vi "FeedbackDecode_20200902.vi"() -> ()   [LabVIEW 2016] (continued)
            n1850 = Bundle By Name(cluster=w1875, "ClearWfs"=TRUE, "SelElect"=w1876, "EventStr"=w1891) -> (w1872:T5)
            n1851 = local read "LoopCnt"() -> (w1889:u64)
            n1852 = call "FeedbackDecode_MLComCtrl.vi"("DecodeClustIn"=w1872, "Mode"=T19."SendEvent") -> ("DecodeClustOut"=w1873:T5)  [unwired: 6 in, 3 out]
            n1853 = local write "DecodeClust"(w1873) -> ()
            n1854 = local write "BaseCnt2"(w1889) -> ()
          }
          event Value Change {
            n1855 = event-data() -> ()  [unwired: 1 in, 6 out]
            n1856 = local read "EncodeClust"() -> (w1921:T9)
            n1857 = call "File Dialog2"("pattern (all files)"="StimParams*.txt") -> ("selected path"=w1924:path, "exists"=w1928:bool, "cancelled"=w1927:bool)  [unwired: 11 in, 1 out]
            n1858 = Unbundle By Name(w1921) -> ("SelPreset"=w1923:bool[], "Sel"=w1922:bool[])
            n1859 = local read "DecodeClust"() -> (w1920:T5)
            n1860 = Not(x=w1927) -> (.not. x?=w1929:bool)
            n1861 = And(x=w1928, y=w1929) -> (x .and. y?=w1925:bool)
            n1862 = case shown="True" w1925 {
              tunnel: w1924 -> [_ w1959]
              tunnel: w1923 -> [_ w1962]
              tunnel: w1922 -> [_ w1961]
              tunnel: w1921 -> [w1932 w1960]
              tunnel: w1920 -> [_ w1945]
              frame False {
                n1863 = Bundle By Name(cluster=w1932, "AdjClust.LoadTable"=FALSE) -> (w1931:T9)
                n1864 = local write "EncodeClust"(w1931) -> ()
              }
              frame True {
                n1865 = call-poly <vilib>:"Read Delimited Spreadsheet.vi"("file path (dialog if empty)"=w1959) -> ("all rows"=w1963:string[][])  [unwired: 9 in, 5 out]
                n1866 = Array Size(array=w1962) -> (size(s)=w1965:i32)
                n1867 = Array Size(array=w1961) -> (size(s)=w1968:i32)
                n1868 = Initialize Array(FALSE, w1965) -> (w1969:bool[])
                n1869 = Initialize Array(FALSE, w1968) -> (w1970:bool[])
                n1870 = Bundle By Name(cluster=w1960, "SelPreset"=w1969, "Sel"=w1970, "ParamsTable"=w1963, "AdjClust.LoadTable"=FALSE) -> (w1957:T9)
                n1871 = Path To String(path=w1959) -> (string=w1955:string)
                n1872 = call "FeedbackDecode_UpdateParamsTable.vi"("StimClustIn"=w1957) -> ("StimClustOut"=w1958:T9)  [unwired: 2 in]
                n1873 = call "FeedbackDecode_Params2UEA.vi"("StimClustIn"=w1958) -> ("StimClustOut"=w1940:T9)  [unwired: 2 in]
                n1874 = local read "LoopCnt"() -> (w1949:u64)
                n1875 = local read "NIPTime"() -> (w1938:dbl)
                n1876 = call "FeedbackDecode_BuildStimCmd.vi"("EncodeClustIn"=w1940) -> ("EncodeClustOut"=w1939:T9, "StimCmd"=w1934:string)  [unwired: 1 in]
                n1877 = Search and Replace String(input string=w1955, search string=":", replace string="@" ("replace string (\"\")")) -> (result string=w1942:string)  [unwired: 5 in, 3 out]
                n1878 = Format Into String(w1949) -> (resulting string=w1946:string)  [unwired: 3 in, 1 out]
                n1879 = call-poly "FeedbackDecode_VariablesToString.vi"("Format"="%0.0f", "ValueIn"=w1938, "FieldName"="NIPTime" ("Key Word")) -> ("StringOut"=w1935:string)  [unwired: 4 in]
                n1880 = local write "EncodeClust"(w1939) -> ()
                n1881 = Concatenate Strings("LoadStimParams:SS.EventID=" ("string"), w1946) -> (w1948:string)
                n1882 = Concatenate Strings(w1948, ";", "SS.StimParamsFile='" ("string"), w1942, "';" ("string"), w1934, w1935) -> (w1944:string)
                n1883 = local write "StimCmd"(w1934) -> ()
                n1884 = Bundle By Name(cluster=w1945, "EventStr"=w1944) -> (w1947:T5)
                n1885 = local read "EventParamsFID"() -> (w1953:refnum<file>)
                n1886 = call "FeedbackDecode_MLComCtrl.vi"("DecodeClustIn"=w1947, "Mode"=T19."SendEvent") -> ()  [unwired: 6 in, 4 out]
                n1887 = call "FeedbackDecode_WriteTextEOL.vi"("text"=w1944, "refnum in"=w1953) -> ()  [unwired: 8 in, 2 out]
              }
            }
          }
          event Value Change {
            n1888 = event-data() -> ()  [unwired: 1 in, 6 out]
            n1889 = local read "EncodeClust"() -> (w1972:T9)
            n1890 = call "File Dialog3"("pattern (all files)"="StimPresets*.txt") -> ("selected path"=w1975:path, "exists"=w1979:bool, "cancelled"=w1978:bool)  [unwired: 11 in, 1 out]
            n1891 = Unbundle By Name(w1972) -> ("SelPreset"=w1974:bool[], "Sel"=w1973:bool[])
            n1892 = local read "DecodeClust"() -> (w1971:T5)
            n1893 = Not(x=w1978) -> (.not. x?=w1980:bool)
            n1894 = And(x=w1979, y=w1980) -> (x .and. y?=w1976:bool)
            n1895 = case shown="True" w1976 {
              tunnel: w1975 -> [_ w2011]
              tunnel: w1974 -> [_ w2014]
              tunnel: w1973 -> [_ w2013]
              tunnel: w1972 -> [w1983 w2012]
              tunnel: w1971 -> [_ w1998]
              frame False {
                n1896 = Bundle By Name(cluster=w1983, "AdjClust.LoadTable"=FALSE) -> (w1982:T9)
                n1897 = local write "EncodeClust"(w1982) -> ()
              }
              frame True {
                n1898 = call-poly <vilib>:"Read Delimited Spreadsheet.vi"("file path (dialog if empty)"=w2011) -> ("all rows"=w2015:string[][])  [unwired: 9 in, 5 out]
                n1899 = Array Size(array=w2014) -> (size(s)=w2017:i32)
                n1900 = Array Size(array=w2013) -> (size(s)=w2020:i32)
                n1901 = Initialize Array(FALSE, w2017) -> (w2021:bool[])
                n1902 = Initialize Array(FALSE, w2020) -> (w2022:bool[])
                n1903 = Bundle By Name(cluster=w2012, "SelPreset"=w2021, "Sel"=w2022, "PresetTable"=w2015, "PresetClust.Load"=FALSE ("AdjClust.LoadTable")) -> (w1986:T9)
                n1904 = Path To String(path=w2011) -> (string=w2008:string)
                n1905 = call "FeedbackDecode_UpdatePresetsTable.vi"("StimClustIn"=w1986) -> ("StimClustOut"=w1985:T9)  [unwired: 2 in]
                n1906 = call "FeedbackDecode_UpdateParamsTable.vi"("StimClustIn"=w1985) -> ("StimClustOut"=w2010:T9)  [unwired: 2 in]
                n1907 = call "FeedbackDecode_Params2UEA.vi"("StimClustIn"=w2010) -> ("StimClustOut"=w1993:T9)  [unwired: 2 in]
                n1908 = local read "LoopCnt"() -> (w2002:u64)
                n1909 = local read "NIPTime"() -> (w1991:dbl)
                n1910 = call "FeedbackDecode_BuildStimCmd.vi"("EncodeClustIn"=w1993) -> ("EncodeClustOut"=w1992:T9, "StimCmd"=w1987:string)  [unwired: 1 in]
                n1911 = Search and Replace String(input string=w2008, search string=":", replace string="@" ("replace string (\"\")")) -> (result string=w1995:string)  [unwired: 5 in, 3 out]
                n1912 = Format Into String(w2002) -> (resulting string=w1999:string)  [unwired: 3 in, 1 out]
                n1913 = call-poly "FeedbackDecode_VariablesToString.vi"("Format"="%0.0f", "ValueIn"=w1991, "FieldName"="NIPTime" ("Key Word")) -> ("StringOut"=w1988:string)  [unwired: 4 in]
                n1914 = local write "EncodeClust"(w1992) -> ()
                n1915 = Concatenate Strings("LoadPresets:SS.EventID=" ("string"), w1999) -> (w2001:string)
                n1916 = Concatenate Strings(w2001, ";", "SS.PresetsFile='" ("string"), w1995, "';" ("string"), w1987, w1988) -> (w1997:string)
                n1917 = local write "StimCmd"(w1987) -> ()
                n1918 = Bundle By Name(cluster=w1998, "EventStr"=w1997) -> (w2000:T5)
                n1919 = local read "EventParamsFID"() -> (w2006:refnum<file>)
                n1920 = call "FeedbackDecode_MLComCtrl.vi"("DecodeClustIn"=w2000, "Mode"=T19."SendEvent") -> ()  [unwired: 6 in, 4 out]
                n1921 = call "FeedbackDecode_WriteTextEOL.vi"("text"=w1997, "refnum in"=w2006) -> ()  [unwired: 8 in, 2 out]
              }
            }
          }
          event Value Change {
            n1922 = event-data() -> ()  [unwired: 1 in, 6 out]
            n1923 = local read "DataPath"() -> (w2027:path)
            n1924 = call "File Dialog"("start path"=w2027) -> ("selected path"=w2024:path, "cancelled"=w2026:bool)  [unwired: 11 in, 2 out]
            n1925 = local read "EncodeClust"() -> (w2025:T9)
            n1926 = local read "DecodeClust"() -> (w2023:T5)
            n1927 = case shown="False" w2026 {
              tunnel: w2025 -> [w2038 w2065]
              tunnel: w2024 -> [w2039 _]
              tunnel: w2023 -> [w2029 _]
              frame False {
                w2048 = "_" ("string")
                n1928 = Strip Path(path=w2039) -> (stripped path=w2046:path, name=w2047:string)
                n1929 = Unbundle By Name(w2029) -> ("DataFolder"=w2036:string)
                n1930 = Get Date/Time In Seconds() -> (seconds since 1Jan1904=w2042:timestamp)
                n1931 = Format Date/Time String(time format string (%c)="%H%M%S", seconds (now)=w2042) -> (date/time string=w2044:string)  [unwired: 1 in]
                n1932 = Concatenate Strings("StimParams_" ("name or relative path"), w2036, w2048, w2047, w2048, w2044, ".txt" ("string")) -> (w2045:string)
                n1933 = Unbundle By Name(w2038) -> ("ParamsTable"=w2040:string[][])
                n1934 = Bundle By Name(cluster=w2038, "AdjClust.SaveTable"=FALSE ("Save")) -> (w2058:T9)
                n1935 = Build Path(base path=w2046, name or relative path=w2045) -> (appended path=w2049:path)
                n1936 = call-poly <vilib>:"Write Delimited Spreadsheet.vi"("file path (dialog if empty)"=w2049, "2D data"=w2040) -> ()  [unwired: 12 in, 2 out]
                n1937 = Path To String(path=w2049) -> (string=w2033:string)
                n1938 = local read "LoopCnt"() -> (w2061:u64)
                n1939 = local write "EncodeClust"(w2058) -> ()
                n1940 = Format Into String(w2061) -> (resulting string=w2050:string)  [unwired: 3 in, 1 out]
                n1941 = Search and Replace String(input string=w2033, search string=":", replace string="@" ("replace string (\"\")")) -> (result string=w2031:string)  [unwired: 5 in, 3 out]
                n1942 = local read "NIPTime"() -> (w2055:dbl)
                n1943 = Concatenate Strings("SaveStimParams:SS.EventID=" ("string"), w2050, ";") -> (w2056:string)
                n1944 = local read "EventParamsFID"() -> (w2064:refnum<file>)
                n1945 = call-poly "FeedbackDecode_VariablesToString.vi"("Format"="%0.0f", "ValueIn"=w2055, "FieldName"="NIPTime" ("Key Word")) -> ("StringOut"=w2052:string)  [unwired: 4 in]
                n1946 = Concatenate Strings(w2056, "SS.StimParamsFile='" ("string"), w2031, "';" ("string"), w2052) -> (w2051:string)
                n1947 = call "FeedbackDecode_WriteTextEOL.vi"("text"=w2051, "refnum in"=w2064) -> ()  [unwired: 8 in, 2 out]
                n1948 = Bundle By Name(cluster=w2029, "EventStr"=w2051) -> (w2060:T5)
                n1949 = call "FeedbackDecode_MLComCtrl.vi"("DecodeClustIn"=w2060, "Mode"=T19."SendEvent") -> ()  [unwired: 6 in, 4 out]
              }
              frame True {
                n1950 = Bundle By Name(cluster=w2065, "AdjClust.SaveTable"=FALSE ("Save")) -> (w2067:T9)
                n1951 = local write "EncodeClust"(w2067) -> ()
              }
            }
          }
          event Value Change {
            n1952 = event-data() -> ()  [unwired: 1 in, 6 out]
            n1953 = local read "DataPath"() -> (w2072:path)
            n1954 = call "File Dialog4"("start path"=w2072) -> ("selected path"=w2069:path, "cancelled"=w2071:bool)  [unwired: 11 in, 2 out]
            n1955 = local read "EncodeClust"() -> (w2070:T9)
            n1956 = local read "DecodeClust"() -> (w2068:T5)
            n1957 = case shown="False" w2071 {
              tunnel: w2070 -> [w2083 w2110]
              tunnel: w2069 -> [w2084 _]
              tunnel: w2068 -> [w2074 _]
              frame False {
                w2093 = "_" ("string")
                n1958 = Strip Path(path=w2084) -> (stripped path=w2091:path, name=w2092:string)
                n1959 = Unbundle By Name(w2074) -> ("DataFolder"=w2081:string)
                n1960 = Get Date/Time In Seconds() -> (seconds since 1Jan1904=w2087:timestamp)
                n1961 = Format Date/Time String(time format string (%c)="%H%M%S", seconds (now)=w2087) -> (date/time string=w2089:string)  [unwired: 1 in]
                n1962 = Concatenate Strings("StimPresets_" ("name or relative path"), w2081, w2093, w2092, w2093, w2089, ".txt" ("string")) -> (w2090:string)
                n1963 = Unbundle By Name(w2083) -> ("PresetTable"=w2085:string[][])
                n1964 = Build Path(base path=w2091, name or relative path=w2090) -> (appended path=w2094:path)
                n1965 = Bundle By Name(cluster=w2083, "PresetClust.Save"=FALSE ("Save")) -> (w2103:T9)
                n1966 = call-poly <vilib>:"Write Delimited Spreadsheet.vi"("file path (dialog if empty)"=w2094, "2D data"=w2085) -> ()  [unwired: 12 in, 2 out]
                n1967 = Path To String(path=w2094) -> (string=w2078:string)
                n1968 = local read "LoopCnt"() -> (w2106:u64)
                n1969 = local write "EncodeClust"(w2103) -> ()
                n1970 = Format Into String(w2106) -> (resulting string=w2095:string)  [unwired: 3 in, 1 out]
                n1971 = Search and Replace String(input string=w2078, search string=":", replace string="@" ("replace string (\"\")")) -> (result string=w2076:string)  [unwired: 5 in, 3 out]
                n1972 = local read "NIPTime"() -> (w2100:dbl)
                n1973 = Concatenate Strings("SavePresets:SS.EventID=" ("string"), w2095, ";") -> (w2101:string)
                n1974 = local read "EventParamsFID"() -> (w2109:refnum<file>)
                n1975 = call-poly "FeedbackDecode_VariablesToString.vi"("Format"="%0.0f", "ValueIn"=w2100, "FieldName"="NIPTime" ("Key Word")) -> ("StringOut"=w2097:string)  [unwired: 4 in]
                n1976 = Concatenate Strings(w2101, "SS.PresetsFile='" ("string"), w2076, "';" ("string"), w2097) -> (w2096:string)
                n1977 = call "FeedbackDecode_WriteTextEOL.vi"("text"=w2096, "refnum in"=w2109) -> ()  [unwired: 8 in, 2 out]
                n1978 = Bundle By Name(cluster=w2074, "EventStr"=w2096) -> (w2105:T5)
                n1979 = call "FeedbackDecode_MLComCtrl.vi"("DecodeClustIn"=w2105, "Mode"=T19."SendEvent") -> ()  [unwired: 6 in, 4 out]
              }
              frame True {
                n1980 = Bundle By Name(cluster=w2110, "AdjClust.SaveTable"=FALSE ("Save")) -> (w2112:T9)
                n1981 = local write "EncodeClust"(w2112) -> ()
              }
            }
          }
          event Value Change {
            n1982 = event-data() -> ()  [unwired: 1 in, 6 out]
            n1983 = local read "EncodeClust"() -> (w2117:T9)
            n1984 = call "FeedbackDecode_Params2Preset.vi"("StimClustIn"=w2117) -> ("StimClustOut"=w2116:T9)  [unwired: 2 in]
            n1985 = local read "LoopCnt"() -> (w2126:u64)
            n1986 = call "FeedbackDecode_UpdateParamsTable.vi"("StimClustIn"=w2116) -> ("StimClustOut"=w2115:T9)  [unwired: 2 in]
            n1987 = call "FeedbackDecode_Params2UEA.vi"("StimClustIn"=w2115) -> ("StimClustOut"=w2114:T9)  [unwired: 2 in]
            n1988 = Format Into String(w2126) -> (resulting string=w2118:string)  [unwired: 3 in, 1 out]
            n1989 = local read "NIPTime"() -> (w2122:dbl)
            n1990 = call "FeedbackDecode_BuildStimCmd.vi"("EncodeClustIn"=w2114) -> ("EncodeClustOut"=w2132:T9, "StimCmd"=w2113:string)  [unwired: 1 in]
            n1991 = local read "EventParamsFID"() -> (w2130:refnum<file>)
            n1992 = Concatenate Strings("UpdateStim:SS.EventID=" ("string"), w2118) -> (w2125:string)
            n1993 = call-poly "FeedbackDecode_VariablesToString.vi"("Format"="%0.0f", "ValueIn"=w2122, "FieldName"="NIPTime" ("Key Word")) -> ("StringOut"=w2119:string)  [unwired: 4 in]
            n1994 = local read "DecodeClust"() -> (w2131:T5)
            n1995 = Concatenate Strings(w2125, ";", w2113, w2119) -> (w2124:string)
            n1996 = call "FeedbackDecode_WriteTextEOL.vi"("text"=w2124, "refnum in"=w2130) -> ()  [unwired: 8 in, 2 out]
            n1997 = Bundle By Name(cluster=w2131, "EventStr"=w2124) -> (w2123:T5)
            n1998 = local write "StimCmd"(w2113) -> ()
            n1999 = local write "EncodeClust"(w2132) -> ()
            n2000 = call "FeedbackDecode_MLComCtrl.vi"("DecodeClustIn"=w2123, "Mode"=T19."SendEvent") -> ()  [unwired: 6 in, 4 out]
          }
          event Value Change {
            n2001 = event-data() -> ("NewVal"=w2139:bool[], "OldVal"=w2138:bool[])  [unwired: 1 in, 4 out]
            n2002 = call "FeedbackDecode_UpdateSelPresets.vi"("OldSelIn"=w2138, "NewSelIn"=w2139) -> ("OldSelOut"=w2137:bool[], "NewSelOut"=w2136:bool[])
            n2003 = Exclusive Or(1:w2137, 2:w2136) -> (0:w2134:bool[])
            n2004 = Or Array Elements(Boolean array=w2136) -> (logical OR=w2135:bool)
            n2005 = case shown="False" w2135 {
              tunnel: w2134 -> [w2143 _]
              frame True {
                n2006 = local read "EncodeClust"() -> (w2144:T9)
                n2007 = Bundle By Name(cluster=w2144, "SelPreset"=w2143) -> (w2142:T9)
                n2008 = call "FeedbackDecode_UpdatePresetsTable.vi"("StimClustIn"=w2142) -> ("StimClustOut"=w2147:T9)  [unwired: 2 in]
                n2009 = local read "LoopCnt"() -> (w2156:u64)
                n2010 = call "FeedbackDecode_UpdateParamsTable.vi"("StimClustIn"=w2147) -> ("StimClustOut"=w2146:T9)  [unwired: 2 in]
                n2011 = call "FeedbackDecode_Params2UEA.vi"("StimClustIn"=w2146) -> ("StimClustOut"=w2145:T9)  [unwired: 2 in]
                n2012 = Format Into String(w2156) -> (resulting string=w2148:string)  [unwired: 3 in, 1 out]
                n2013 = local read "NIPTime"() -> (w2152:dbl)
                n2014 = call "FeedbackDecode_BuildStimCmd.vi"("EncodeClustIn"=w2145) -> ("EncodeClustOut"=w2162:T9, "StimCmd"=w2141:string)  [unwired: 1 in]
                n2015 = local read "EventParamsFID"() -> (w2160:refnum<file>)
                n2016 = Concatenate Strings("UpdateStim:SS.EventID=" ("string"), w2148) -> (w2155:string)
                n2017 = call-poly "FeedbackDecode_VariablesToString.vi"("Format"="%0.0f", "ValueIn"=w2152, "FieldName"="NIPTime" ("Key Word")) -> ("StringOut"=w2149:string)  [unwired: 4 in]
                n2018 = local read "DecodeClust"() -> (w2161:T5)
                n2019 = Concatenate Strings(w2155, ";", w2141, w2149) -> (w2154:string)
                n2020 = call "FeedbackDecode_WriteTextEOL.vi"("text"=w2154, "refnum in"=w2160) -> ()  [unwired: 8 in, 2 out]
                n2021 = Bundle By Name(cluster=w2161, "EventStr"=w2154) -> (w2153:T5)
                n2022 = local write "StimCmd"(w2141) -> ()
                n2023 = local write "EncodeClust"(w2162) -> ()
                n2024 = call "FeedbackDecode_MLComCtrl.vi"("DecodeClustIn"=w2153, "Mode"=T19."SendEvent") -> ()  [unwired: 6 in, 4 out]
              }
              frame False {
                n2025 = local read "EncodeClust"() -> (w2165:T9)
                n2026 = Unbundle By Name(w2165) -> ("Sel"=w2167:bool[])
                n2027 = Array Size(array=w2167) -> (size(s)=w2168:i32)
                n2028 = Initialize Array(FALSE, w2168) -> (w2166:bool[])
                n2029 = Bundle By Name(cluster=w2165, "Sel"=w2166) -> (w2164:T9)
                n2030 = local read "LoopCnt"() -> (w2180:u64)
                n2031 = call "FeedbackDecode_UpdateParamsTable.vi"("StimClustIn"=w2164) -> ("StimClustOut"=w2171:T9)  [unwired: 2 in]
                n2032 = call "FeedbackDecode_Params2UEA.vi"("StimClustIn"=w2171) -> ("StimClustOut"=w2170:T9)  [unwired: 2 in]
                n2033 = Format Into String(w2180) -> (resulting string=w2172:string)  [unwired: 3 in, 1 out]
                n2034 = local read "NIPTime"() -> (w2176:dbl)
                n2035 = call "FeedbackDecode_BuildStimCmd.vi"("EncodeClustIn"=w2170) -> ("EncodeClustOut"=w2186:T9, "StimCmd"=w2163:string)  [unwired: 1 in]
                n2036 = local read "EventParamsFID"() -> (w2184:refnum<file>)
                n2037 = Concatenate Strings("UpdateStim:SS.EventID=" ("string"), w2172) -> (w2179:string)
                n2038 = call-poly "FeedbackDecode_VariablesToString.vi"("Format"="%0.0f", "ValueIn"=w2176, "FieldName"="NIPTime" ("Key Word")) -> ("StringOut"=w2173:string)  [unwired: 4 in]
                n2039 = local read "DecodeClust"() -> (w2185:T5)
                n2040 = Concatenate Strings(w2179, ";", w2163, w2173) -> (w2178:string)
                n2041 = call "FeedbackDecode_WriteTextEOL.vi"("text"=w2178, "refnum in"=w2184) -> ()  [unwired: 8 in, 2 out]
                n2042 = Bundle By Name(cluster=w2185, "EventStr"=w2178) -> (w2177:T5)
                n2043 = local write "StimCmd"(w2163) -> ()
                n2044 = local write "EncodeClust"(w2186) -> ()
                n2045 = call "FeedbackDecode_MLComCtrl.vi"("DecodeClustIn"=w2177, "Mode"=T19."SendEvent") -> ()  [unwired: 6 in, 4 out]
              }
            }
          }
          event Value Change {
            n2046 = event-data() -> ()  [unwired: 1 in, 6 out]
            n2047 = local read "EncodeClust"() -> (w2191:T9)
            n2048 = call "FeedbackDecode_UEA2Params.vi"("StimClustIn"=w2191) -> ("StimClustOut"=w2190:T9)  [unwired: 2 in]
            n2049 = local read "LoopCnt"() -> (w2200:u64)
            n2050 = call "FeedbackDecode_UpdateParamsTable.vi"("StimClustIn"=w2190) -> ("StimClustOut"=w2189:T9)  [unwired: 2 in]
            n2051 = call "FeedbackDecode_Params2Preset.vi"("StimClustIn"=w2189) -> ("StimClustOut"=w2188:T9)  [unwired: 2 in]
            n2052 = Format Into String(w2200) -> (resulting string=w2192:string)  [unwired: 3 in, 1 out]
            n2053 = local read "NIPTime"() -> (w2196:dbl)
            n2054 = call "FeedbackDecode_BuildStimCmd.vi"("EncodeClustIn"=w2188) -> ("EncodeClustOut"=w2206:T9, "StimCmd"=w2187:string)  [unwired: 1 in]
            n2055 = local read "EventParamsFID"() -> (w2204:refnum<file>)
            n2056 = Concatenate Strings("UpdateStim:SS.EventID=" ("string"), w2192) -> (w2199:string)
            n2057 = call-poly "FeedbackDecode_VariablesToString.vi"("Format"="%0.0f", "ValueIn"=w2196, "FieldName"="NIPTime" ("Key Word")) -> ("StringOut"=w2193:string)  [unwired: 4 in]
            n2058 = local read "DecodeClust"() -> (w2205:T5)
            n2059 = Concatenate Strings(w2199, ";", w2187, w2193) -> (w2198:string)
            n2060 = call "FeedbackDecode_WriteTextEOL.vi"("text"=w2198, "refnum in"=w2204) -> ()  [unwired: 8 in, 2 out]
            n2061 = Bundle By Name(cluster=w2205, "EventStr"=w2198) -> (w2197:T5)
            n2062 = local write "StimCmd"(w2187) -> ()
            n2063 = local write "EncodeClust"(w2206) -> ()
            n2064 = call "FeedbackDecode_MLComCtrl.vi"("DecodeClustIn"=w2197, "Mode"=T19."SendEvent") -> ()  [unwired: 6 in, 4 out]
          }
          event Value Change {
            n2065 = event-data() -> ()  [unwired: 1 in, 6 out]
            n2066 = local read "EncodeClust"() -> (w2213:T9)
            n2067 = call "FeedbackDecode_AdjParamsTable.vi"("StimClustIn"=w2213, "Mode"=enum16{"Set", "Add", "Sub"}."Set") -> ("StimClustOut"=w2211:T9)  [unwired: 1 in]
            n2068 = Bundle By Name(cluster=w2211, "AdjClust.Set"=FALSE) -> (w2209:T9)
            n2069 = local read "LoopCnt"() -> (w2223:u64)
            n2070 = call "FeedbackDecode_Params2Preset.vi"("StimClustIn"=w2209) -> ("StimClustOut"=w2214:T9)  [unwired: 2 in]
            n2071 = Format Into String(w2223) -> (resulting string=w2215:string)  [unwired: 3 in, 1 out]
            n2072 = local read "NIPTime"() -> (w2219:dbl)
            n2073 = call "FeedbackDecode_BuildStimCmd.vi"("EncodeClustIn"=w2214) -> ("EncodeClustOut"=w2229:T9, "StimCmd"=w2208:string)  [unwired: 1 in]
            n2074 = local read "EventParamsFID"() -> (w2227:refnum<file>)
            n2075 = Concatenate Strings("UpdateStim:SS.EventID=" ("string"), w2215) -> (w2222:string)
            n2076 = call-poly "FeedbackDecode_VariablesToString.vi"("Format"="%0.0f", "ValueIn"=w2219, "FieldName"="NIPTime" ("Key Word")) -> ("StringOut"=w2216:string)  [unwired: 4 in]
            n2077 = local read "DecodeClust"() -> (w2228:T5)
            n2078 = Concatenate Strings(w2222, ";", w2208, w2216) -> (w2221:string)
            n2079 = call "FeedbackDecode_WriteTextEOL.vi"("text"=w2221, "refnum in"=w2227) -> ()  [unwired: 8 in, 2 out]
            n2080 = Bundle By Name(cluster=w2228, "EventStr"=w2221) -> (w2220:T5)
            n2081 = local write "StimCmd"(w2208) -> ()
            n2082 = local write "EncodeClust"(w2229) -> ()
            n2083 = call "FeedbackDecode_MLComCtrl.vi"("DecodeClustIn"=w2220, "Mode"=T19."SendEvent") -> ()  [unwired: 6 in, 4 out]
          }
          event Value Change {
            n2084 = event-data() -> ()  [unwired: 1 in, 6 out]
            n2085 = local read "EncodeClust"() -> (w2236:T9)
            n2086 = call "FeedbackDecode_AdjParamsTable.vi"("StimClustIn"=w2236, "Mode"=enum16{"Set", "Add", "Sub"}."Add") -> ("StimClustOut"=w2234:T9)  [unwired: 1 in]
            n2087 = Bundle By Name(cluster=w2234, "AdjClust.Add"=FALSE ("AdjClust.Set")) -> (w2232:T9)
            n2088 = local read "LoopCnt"() -> (w2246:u64)
            n2089 = call "FeedbackDecode_Params2Preset.vi"("StimClustIn"=w2232) -> ("StimClustOut"=w2237:T9)  [unwired: 2 in]
            n2090 = Format Into String(w2246) -> (resulting string=w2238:string)  [unwired: 3 in, 1 out]
            n2091 = local read "NIPTime"() -> (w2242:dbl)
            n2092 = call "FeedbackDecode_BuildStimCmd.vi"("EncodeClustIn"=w2237) -> ("EncodeClustOut"=w2252:T9, "StimCmd"=w2231:string)  [unwired: 1 in]
            n2093 = local read "EventParamsFID"() -> (w2250:refnum<file>)
            n2094 = Concatenate Strings("UpdateStim:SS.EventID=" ("string"), w2238) -> (w2245:string)
            n2095 = call-poly "FeedbackDecode_VariablesToString.vi"("Format"="%0.0f", "ValueIn"=w2242, "FieldName"="NIPTime" ("Key Word")) -> ("StringOut"=w2239:string)  [unwired: 4 in]
            n2096 = local read "DecodeClust"() -> (w2251:T5)
            n2097 = Concatenate Strings(w2245, ";", w2231, w2239) -> (w2244:string)
            n2098 = call "FeedbackDecode_WriteTextEOL.vi"("text"=w2244, "refnum in"=w2250) -> ()  [unwired: 8 in, 2 out]
            n2099 = Bundle By Name(cluster=w2251, "EventStr"=w2244) -> (w2243:T5)
            n2100 = local write "StimCmd"(w2231) -> ()
            n2101 = local write "EncodeClust"(w2252) -> ()
            n2102 = call "FeedbackDecode_MLComCtrl.vi"("DecodeClustIn"=w2243, "Mode"=T19."SendEvent") -> ()  [unwired: 6 in, 4 out]
          }
          event Value Change {
            n2103 = event-data() -> ()  [unwired: 1 in, 6 out]
            n2104 = local read "EncodeClust"() -> (w2259:T9)
            n2105 = call "FeedbackDecode_AdjParamsTable.vi"("StimClustIn"=w2259, "Mode"=enum16{"Set", "Add", "Sub"}."Sub") -> ("StimClustOut"=w2257:T9)  [unwired: 1 in]
            n2106 = Bundle By Name(cluster=w2257, "AdjClust.Sub"=FALSE ("AdjClust.Set")) -> (w2255:T9)
            n2107 = local read "LoopCnt"() -> (w2269:u64)
            n2108 = call "FeedbackDecode_Params2Preset.vi"("StimClustIn"=w2255) -> ("StimClustOut"=w2260:T9)  [unwired: 2 in]
            n2109 = Format Into String(w2269) -> (resulting string=w2261:string)  [unwired: 3 in, 1 out]
            n2110 = local read "NIPTime"() -> (w2265:dbl)
            n2111 = call "FeedbackDecode_BuildStimCmd.vi"("EncodeClustIn"=w2260) -> ("EncodeClustOut"=w2275:T9, "StimCmd"=w2254:string)  [unwired: 1 in]
            n2112 = local read "EventParamsFID"() -> (w2273:refnum<file>)
            n2113 = Concatenate Strings("UpdateStim:SS.EventID=" ("string"), w2261) -> (w2268:string)
            n2114 = call-poly "FeedbackDecode_VariablesToString.vi"("Format"="%0.0f", "ValueIn"=w2265, "FieldName"="NIPTime" ("Key Word")) -> ("StringOut"=w2262:string)  [unwired: 4 in]
            n2115 = local read "DecodeClust"() -> (w2274:T5)
            n2116 = Concatenate Strings(w2268, ";", w2254, w2262) -> (w2267:string)
            n2117 = call "FeedbackDecode_WriteTextEOL.vi"("text"=w2267, "refnum in"=w2273) -> ()  [unwired: 8 in, 2 out]
            n2118 = Bundle By Name(cluster=w2274, "EventStr"=w2267) -> (w2266:T5)
            n2119 = local write "StimCmd"(w2254) -> ()
            n2120 = local write "EncodeClust"(w2275) -> ()
            n2121 = call "FeedbackDecode_MLComCtrl.vi"("DecodeClustIn"=w2266, "Mode"=T19."SendEvent") -> ()  [unwired: 6 in, 4 out]
          }
          event Value Change {
            n2122 = event-data() -> ()  [unwired: 1 in, 6 out]
            n2123 = local read "EncodeClust"() -> (w2289:T9)
            n2124 = Unbundle By Name(w2289) -> ("Sel"=w2282:bool[], "ParamsTable"=w2283:string[][], "SelPreset"=w2287:bool[])
            n2125 = while {
              shift-right: [w2315] -> w2281
              shift-left: w2282 -> [w2314]
              shift-right: [w2310] -> w2280
              shift-left: w2283 -> [w2311]
              stop <- w2308 stop-if-true
              n2126 = Search 1D Array(1D array=w2314, element=TRUE) -> (index of element=w2309:i32)  [unwired: 1 in]
              n2127 = Less Than 0?(x=w2309) -> (x < 0?=w2308:bool)
              n2128 = Delete From Array(array=w2314, length=1, index=w2309) -> (array with subset deleted=w2315:bool[])  [unwired: 1 out]
              n2129 = Delete From Array(array=w2311, length=1, index (row)=w2309) -> (array with subset deleted=w2310:string[][])  [unwired: 1 in, 1 out]
            }
            n2130 = Array Size(array=w2287) -> (size(s)=w2285:i32)
            n2131 = Initialize Array(FALSE, w2285) -> (w2288:bool[])
            n2132 = Bundle By Name(cluster=w2289, "Sel"=w2281, "ParamsTable"=w2280, "AdjClust.DeleteSel"=FALSE, "SelPreset"=w2288) -> (w2279:T9)
            n2133 = local read "LoopCnt"() -> (w2299:u64)
            n2134 = call "FeedbackDecode_UpdateParamsTable.vi"("StimClustIn"=w2279) -> ("StimClustOut"=w2278:T9)  [unwired: 2 in]
            n2135 = call "FeedbackDecode_Params2UEA.vi"("StimClustIn"=w2278) -> ("StimClustOut"=w2290:T9)  [unwired: 2 in]
            n2136 = Format Into String(w2299) -> (resulting string=w2291:string)  [unwired: 3 in, 1 out]
            n2137 = local read "NIPTime"() -> (w2295:dbl)
            n2138 = call "FeedbackDecode_BuildStimCmd.vi"("EncodeClustIn"=w2290) -> ("EncodeClustOut"=w2305:T9, "StimCmd"=w2277:string)  [unwired: 1 in]
            n2139 = local read "EventParamsFID"() -> (w2303:refnum<file>)
            n2140 = Concatenate Strings("DelStimParam:SS.EventID=" ("string"), w2291) -> (w2298:string)
            n2141 = call-poly "FeedbackDecode_VariablesToString.vi"("Format"="%0.0f", "ValueIn"=w2295, "FieldName"="NIPTime" ("Key Word")) -> ("StringOut"=w2292:string)  [unwired: 4 in]
            n2142 = local read "DecodeClust"() -> (w2304:T5)
            n2143 = Concatenate Strings(w2298, ";", w2277, w2292) -> (w2297:string)
            n2144 = call "FeedbackDecode_WriteTextEOL.vi"("text"=w2297, "refnum in"=w2303) -> ()  [unwired: 8 in, 2 out]
            n2145 = Bundle By Name(cluster=w2304, "EventStr"=w2297) -> (w2296:T5)
            n2146 = local write "StimCmd"(w2277) -> ()
            n2147 = local write "EncodeClust"(w2305) -> ()
            n2148 = call "FeedbackDecode_MLComCtrl.vi"("DecodeClustIn"=w2296, "Mode"=T19."SendEvent") -> ()  [unwired: 6 in, 4 out]
          }
          event Value Change {
            n2149 = event-data() -> ()  [unwired: 1 in, 6 out]
            n2150 = local read "EncodeClust"() -> (w2329:T9)
            n2151 = Unbundle By Name(w2329) -> ("SelPreset"=w2322:bool[], "PresetTable"=w2323:string[][], "Sel"=w2327:bool[])
            n2152 = while {
              shift-right: [w2355] -> w2321
              shift-left: w2322 -> [w2354]
              shift-right: [w2350] -> w2320
              shift-left: w2323 -> [w2351]
              stop <- w2348 stop-if-true
              n2153 = Search 1D Array(1D array=w2354, element=TRUE) -> (index of element=w2349:i32)  [unwired: 1 in]
              n2154 = Less Than 0?(x=w2349) -> (x < 0?=w2348:bool)
              n2155 = Delete From Array(array=w2354, length=1, index=w2349) -> (array with subset deleted=w2355:bool[])  [unwired: 1 out]
              n2156 = Delete From Array(array=w2351, length=1, index (row)=w2349) -> (array with subset deleted=w2350:string[][])  [unwired: 1 in, 1 out]
            }
            n2157 = Array Size(array=w2327) -> (size(s)=w2325:i32)
            n2158 = Initialize Array(FALSE, w2325) -> (w2328:bool[])
            n2159 = Bundle By Name(cluster=w2329, "SelPreset"=w2321, "PresetTable"=w2320, "PresetClust.Del"=FALSE ("AdjClust.DeleteSel"), "Sel"=w2328) -> (w2317:T9)
            n2160 = call "FeedbackDecode_UpdatePresetsTable.vi"("StimClustIn"=w2317) -> ("StimClustOut"=w2316:T9)  [unwired: 2 in]
            n2161 = local read "LoopCnt"() -> (w2339:u64)
            n2162 = call "FeedbackDecode_UpdateParamsTable.vi"("StimClustIn"=w2316) -> ("StimClustOut"=w2319:T9)  [unwired: 2 in]
            n2163 = call "FeedbackDecode_Params2UEA.vi"("StimClustIn"=w2319) -> ("StimClustOut"=w2330:T9)  [unwired: 2 in]
            n2164 = Format Into String(w2339) -> (resulting string=w2331:string)  [unwired: 3 in, 1 out]
            n2165 = local read "NIPTime"() -> (w2335:dbl)
            n2166 = call "FeedbackDecode_BuildStimCmd.vi"("EncodeClustIn"=w2330) -> ("EncodeClustOut"=w2345:T9, "StimCmd"=w2318:string)  [unwired: 1 in]
            n2167 = local read "EventParamsFID"() -> (w2343:refnum<file>)
            n2168 = Concatenate Strings("DelPreset:SS.EventID=" ("string"), w2331) -> (w2338:string)
            n2169 = call-poly "FeedbackDecode_VariablesToString.vi"("Format"="%0.0f", "ValueIn"=w2335, "FieldName"="NIPTime" ("Key Word")) -> ("StringOut"=w2332:string)  [unwired: 4 in]
            n2170 = local read "DecodeClust"() -> (w2344:T5)
            n2171 = Concatenate Strings(w2338, ";", w2318, w2332) -> (w2337:string)
            n2172 = call "FeedbackDecode_WriteTextEOL.vi"("text"=w2337, "refnum in"=w2343) -> ()  [unwired: 8 in, 2 out]
            n2173 = Bundle By Name(cluster=w2344, "EventStr"=w2337) -> (w2336:T5)
            n2174 = local write "StimCmd"(w2318) -> ()
            n2175 = local write "EncodeClust"(w2345) -> ()
            n2176 = call "FeedbackDecode_MLComCtrl.vi"("DecodeClustIn"=w2336, "Mode"=T19."SendEvent") -> ()  [unwired: 6 in, 4 out]
          }
          event Value Change {
            n2177 = event-data() -> ()  [unwired: 1 in, 6 out]
            n2178 = local read "EncodeClust"() -> (w2366:T9)
            n2179 = Unbundle By Name(w2366) -> ("SelPreset"=w2362:bool[])
            n2180 = Array Size(array=w2362) -> (size(s)=w2364:i32)
            n2181 = Initialize Array(FALSE, w2364) -> (w2365:bool[])
            n2182 = Bundle By Name(cluster=w2366, "ParamsTable"=string[][] [], "Sel"=bool[] [], "UEAArray"=T25 [{"Boolean 1"=FALSE, "Boolean 2"=FALSE, "Boolean 3"=FALSE, "Boolean 4"=FALSE, "Boolean 5"=FALSE, "Boolean 6"=FALSE, "Boolean 7"=FALSE, "Boolean 8"=FALSE, "Boolean 9"=FALSE, "Boolean 10"=FALSE, "Boolean 11"=FALSE, "Boolean 12"=FALSE, "Boolean 13"=FALSE, "Boolean 14"=FALSE, "Boolean 15"=FALSE, "Boolean 16"=FALSE, "Boolean 17"=FALSE, "Boolean 18"=FALSE, "Boolean 19"=FALSE, "Boolean 20"=FALSE, "Boolean 21"=FALSE, "Boolean 22"=FALSE, "Boolean 23"=FALSE, "Boolean 24"=FALSE, "Boolean 25"=FALSE, "Boolean 26"=FALSE, "Boolean 27"=FALSE, "Boolean 28"=FALSE, "Boolean 29"=FALSE, "Boolean 30"=FALSE, "Boolean 31"=FALSE, "Boolean 32"=FALSE, "Boolean 33"=FALSE, "Boolean 34"=FALSE, "Boolean 35"=FALSE, "Boolean 36"=FALSE, "Boolean 37"=FALSE, "Boolean 38"=FALSE, "Boolean 39"=FALSE, "Boolean 40"=FALSE, "Boolean 41"=FALSE, "Boolean 42"=FALSE, "Boolean 43"=FALSE, "Boolean 44"=FALSE, "Boolean 45"=FALSE, "Boolean 46"=FALSE, "Boolean 47"=FALSE, "Boolean 48"=FALSE, "Boolean 49"=FALSE, "Boolean 50"=FALSE, "Boolean 51"=FALSE, "Boolean 52"=FALSE, "Boolean 53"=FALSE, "Boolean 54"=FALSE, "Boolean 55"=FALSE, "Boolean 56"=FALSE, "Boolean 57"=FALSE, "Boolean 58"=FALSE, "Boolean 59"=FALSE, "Boolean 60"=FALSE, "Boolean 61"=FALSE, "Boolean 62"=FALSE, "Boolean 63"=FALSE, "Boolean 64"=FALSE, "Boolean 65"=FALSE, "Boolean 66"=FALSE, "Boolean 67"=FALSE, "Boolean 68"=FALSE, "Boolean 69"=FALSE, "Boolean 70"=FALSE, "Boolean 71"=FALSE, "Boolean 72"=FALSE, "Boolean 73"=FALSE, "Boolean 74"=FALSE, "Boolean 75"=FALSE, "Boolean 76"=FALSE, "Boolean 77"=FALSE, "Boolean 78"=FALSE, "Boolean 79"=FALSE, "Boolean 80"=FALSE, "Boolean 81"=FALSE, "Boolean 82"=FALSE, "Boolean 83"=FALSE, "Boolean 84"=FALSE, "Boolean 85"=FALSE, "Boolean 86"=FALSE, "Boolean 87"=FALSE, "Boolean 88"=FALSE, "Boolean 89"=FALSE, "Boolean 90"=FALSE, "Boolean 91"=FALSE, "Boolean 92"=FALSE, "Boolean 93"=FALSE, "Boolean 94"=FALSE, "Boolean 95"=FALSE, "Boolean 96"=FALSE, "Boolean 97"=FALSE, "Boolean 98"=FALSE, "Boolean 99"=FALSE, "Boolean 100"=FALSE}, {"Boolean 1"=FALSE, "Boolean 2"=FALSE, "Boolean 3"=FALSE, "Boolean 4"=FALSE, "Boolean 5"=FALSE, "Boolean 6"=FALSE, "Boolean 7"=FALSE, "Boolean 8"=FALSE, "Boolean 9"=FALSE, "Boolean 10"=FALSE, "Boolean 11"=FALSE, "Boolean 12"=FALSE, "Boolean 13"=FALSE, "Boolean 14"=FALSE, "Boolean 15"=FALSE, "Boolean 16"=FALSE, "Boolean 17"=FALSE, "Boolean 18"=FALSE, "Boolean 19"=FALSE, "Boolean 20"=FALSE, "Boolean 21"=FALSE, "Boolean 22"=FALSE, "Boolean 23"=FALSE, "Boolean 24"=FALSE, "Boolean 25"=FALSE, "Boolean 26"=FALSE, "Boolean 27"=FALSE, "Boolean 28"=FALSE, "Boolean 29"=FALSE, "Boolean 30"=FALSE, "Boolean 31"=FALSE, "Boolean 32"=FALSE, "Boolean 33"=FALSE, "Boolean 34"=FALSE, "Boolean 35"=FALSE, "Boolean 36"=FALSE, "Boolean 37"=FALSE, "Boolean 38"=FALSE, "Boolean 39"=FALSE, "Boolean 40"=FALSE, "Boolean 41"=FALSE, "Boolean 42"=FALSE, "Boolean 43"=FALSE, "Boolean 44"=FALSE, "Boolean 45"=FALSE, "Boolean 46"=FALSE, "Boolean 47"=FALSE, "Boolean 48"=FALSE, "Boolean 49"=FALSE, "Boolean 50"=FALSE, "Boolean 51"=FALSE, "Boolean 52"=FALSE, "Boolean 53"=FALSE, "Boolean 54"=FALSE, "Boolean 55"=FALSE, "Boolean 56"=FALSE, "Boolean 57"=FALSE, "Boolean 58"=FALSE, "Boolean 59"=FALSE, "Boolean 60"=FALSE, "Boolean 61"=FALSE, "Boolean 62"=FALSE, "Boolean 63"=FALSE, "Boolean 64"=FALSE, "Boolean 65"=FALSE, "Boolean 66"=FALSE, "Boolean 67"=FALSE, "Boolean 68"=FALSE, "Boolean 69"=FALSE, "Boolean 70"=FALSE, "Boolean 71"=FALSE, "Boolean 72"=FALSE, "Boolean 73"=FALSE, "Boolean 74"=FALSE, "Boolean 75"=FALSE, "Boolean 76"=FALSE, "Boolean 77"=FALSE, "Boolean 78"=FALSE, "Boolean 79"=FALSE, "Boolean 80"=FALSE, "Boolean 81"=FALSE, "Boolean 82"=FALSE, "Boolean 83"=FALSE, "Boolean 84"=FALSE, "Boolean 85"=FALSE, "Boolean 86"=FALSE, "Boolean 87"=FALSE, "Boolean 88"=FALSE, "Boolean 89"=FALSE, "Boolean 90"=FALSE, "Boolean 91"=FALSE, "Boolean 92"=FALSE, "Boolean 93"=FALSE, "Boolean 94"=FALSE, "Boolean 95"=FALSE, "Boolean 96"=FALSE, "Boolean 97"=FALSE, "Boolean 98"=FALSE, "Boolean 99"=FALSE, "Boolean 100"=FALSE}], "AdjClust.ClearTable"=FALSE, "SelPreset"=w2365) -> (w2357:T9)
            n2183 = local read "LoopCnt"() -> (w2377:u64)
            n2184 = call "FeedbackDecode_UpdateParamsTable.vi"("StimClustIn"=w2357) -> ("StimClustOut"=w2367:T9)  [unwired: 2 in]
            n2185 = call "FeedbackDecode_Params2UEA.vi"("StimClustIn"=w2367) -> ("StimClustOut"=w2368:T9)  [unwired: 2 in]
            n2186 = Format Into String(w2377) -> (resulting string=w2369:string)  [unwired: 3 in, 1 out]
            n2187 = local read "NIPTime"() -> (w2373:dbl)
            n2188 = call "FeedbackDecode_BuildStimCmd.vi"("EncodeClustIn"=w2368) -> ("EncodeClustOut"=w2383:T9, "StimCmd"=w2356:string)  [unwired: 1 in]
            n2189 = local read "EventParamsFID"() -> (w2381:refnum<file>)
            n2190 = Concatenate Strings("ClearStimParams:SS.EventID=" ("string"), w2369) -> (w2376:string)
            n2191 = call-poly "FeedbackDecode_VariablesToString.vi"("Format"="%0.0f", "ValueIn"=w2373, "FieldName"="NIPTime" ("Key Word")) -> ("StringOut"=w2370:string)  [unwired: 4 in]
            n2192 = local read "DecodeClust"() -> (w2382:T5)
            n2193 = Concatenate Strings(w2376, ";", w2356, w2370) -> (w2375:string)
            n2194 = call "FeedbackDecode_WriteTextEOL.vi"("text"=w2375, "refnum in"=w2381) -> ()  [unwired: 8 in, 2 out]
            n2195 = Bundle By Name(cluster=w2382, "EventStr"=w2375) -> (w2374:T5)
            n2196 = local write "StimCmd"(w2356) -> ()
            n2197 = local write "EncodeClust"(w2383) -> ()
            n2198 = call "FeedbackDecode_MLComCtrl.vi"("DecodeClustIn"=w2374, "Mode"=T19."SendEvent") -> ()  [unwired: 6 in, 4 out]
          }
          event Value Change {
            n2199 = event-data() -> ()  [unwired: 1 in, 6 out]
            n2200 = local read "EncodeClust"() -> (w2396:T9)
            n2201 = Unbundle By Name(w2396) -> ("Sel"=w2392:bool[])
            n2202 = Array Size(array=w2392) -> (size(s)=w2394:i32)
            n2203 = Initialize Array(FALSE, w2394) -> (w2395:bool[])
            n2204 = Bundle By Name(cluster=w2396, "PresetTable"=string[][] [] ("ParamsTable"), "SelPreset"=bool[] [] ("Sel"), "UEAArray"=T25 [{"Boolean 1"=FALSE, "Boolean 2"=FALSE, "Boolean 3"=FALSE, "Boolean 4"=FALSE, "Boolean 5"=FALSE, "Boolean 6"=FALSE, "Boolean 7"=FALSE, "Boolean 8"=FALSE, "Boolean 9"=FALSE, "Boolean 10"=FALSE, "Boolean 11"=FALSE, "Boolean 12"=FALSE, "Boolean 13"=FALSE, "Boolean 14"=FALSE, "Boolean 15"=FALSE, "Boolean 16"=FALSE, "Boolean 17"=FALSE, "Boolean 18"=FALSE, "Boolean 19"=FALSE, "Boolean 20"=FALSE, "Boolean 21"=FALSE, "Boolean 22"=FALSE, "Boolean 23"=FALSE, "Boolean 24"=FALSE, "Boolean 25"=FALSE, "Boolean 26"=FALSE, "Boolean 27"=FALSE, "Boolean 28"=FALSE, "Boolean 29"=FALSE, "Boolean 30"=FALSE, "Boolean 31"=FALSE, "Boolean 32"=FALSE, "Boolean 33"=FALSE, "Boolean 34"=FALSE, "Boolean 35"=FALSE, "Boolean 36"=FALSE, "Boolean 37"=FALSE, "Boolean 38"=FALSE, "Boolean 39"=FALSE, "Boolean 40"=FALSE, "Boolean 41"=FALSE, "Boolean 42"=FALSE, "Boolean 43"=FALSE, "Boolean 44"=FALSE, "Boolean 45"=FALSE, "Boolean 46"=FALSE, "Boolean 47"=FALSE, "Boolean 48"=FALSE, "Boolean 49"=FALSE, "Boolean 50"=FALSE, "Boolean 51"=FALSE, "Boolean 52"=FALSE, "Boolean 53"=FALSE, "Boolean 54"=FALSE, "Boolean 55"=FALSE, "Boolean 56"=FALSE, "Boolean 57"=FALSE, "Boolean 58"=FALSE, "Boolean 59"=FALSE, "Boolean 60"=FALSE, "Boolean 61"=FALSE, "Boolean 62"=FALSE, "Boolean 63"=FALSE, "Boolean 64"=FALSE, "Boolean 65"=FALSE, "Boolean 66"=FALSE, "Boolean 67"=FALSE, "Boolean 68"=FALSE, "Boolean 69"=FALSE, "Boolean 70"=FALSE, "Boolean 71"=FALSE, "Boolean 72"=FALSE, "Boolean 73"=FALSE, "Boolean 74"=FALSE, "Boolean 75"=FALSE, "Boolean 76"=FALSE, "Boolean 77"=FALSE, "Boolean 78"=FALSE, "Boolean 79"=FALSE, "Boolean 80"=FALSE, "Boolean 81"=FALSE, "Boolean 82"=FALSE, "Boolean 83"=FALSE, "Boolean 84"=FALSE, "Boolean 85"=FALSE, "Boolean 86"=FALSE, "Boolean 87"=FALSE, "Boolean 88"=FALSE, "Boolean 89"=FALSE, "Boolean 90"=FALSE, "Boolean 91"=FALSE, "Boolean 92"=FALSE, "Boolean 93"=FALSE, "Boolean 94"=FALSE, "Boolean 95"=FALSE, "Boolean 96"=FALSE, "Boolean 97"=FALSE, "Boolean 98"=FALSE, "Boolean 99"=FALSE, "Boolean 100"=FALSE}, {"Boolean 1"=FALSE, "Boolean 2"=FALSE, "Boolean 3"=FALSE, "Boolean 4"=FALSE, "Boolean 5"=FALSE, "Boolean 6"=FALSE, "Boolean 7"=FALSE, "Boolean 8"=FALSE, "Boolean 9"=FALSE, "Boolean 10"=FALSE, "Boolean 11"=FALSE, "Boolean 12"=FALSE, "Boolean 13"=FALSE, "Boolean 14"=FALSE, "Boolean 15"=FALSE, "Boolean 16"=FALSE, "Boolean 17"=FALSE, "Boolean 18"=FALSE, "Boolean 19"=FALSE, "Boolean 20"=FALSE, "Boolean 21"=FALSE, "Boolean 22"=FALSE, "Boolean 23"=FALSE, "Boolean 24"=FALSE, "Boolean 25"=FALSE, "Boolean 26"=FALSE, "Boolean 27"=FALSE, "Boolean 28"=FALSE, "Boolean 29"=FALSE, "Boolean 30"=FALSE, "Boolean 31"=FALSE, "Boolean 32"=FALSE, "Boolean 33"=FALSE, "Boolean 34"=FALSE, "Boolean 35"=FALSE, "Boolean 36"=FALSE, "Boolean 37"=FALSE, "Boolean 38"=FALSE, "Boolean 39"=FALSE, "Boolean 40"=FALSE, "Boolean 41"=FALSE, "Boolean 42"=FALSE, "Boolean 43"=FALSE, "Boolean 44"=FALSE, "Boolean 45"=FALSE, "Boolean 46"=FALSE, "Boolean 47"=FALSE, "Boolean 48"=FALSE, "Boolean 49"=FALSE, "Boolean 50"=FALSE, "Boolean 51"=FALSE, "Boolean 52"=FALSE, "Boolean 53"=FALSE, "Boolean 54"=FALSE, "Boolean 55"=FALSE, "Boolean 56"=FALSE, "Boolean 57"=FALSE, "Boolean 58"=FALSE, "Boolean 59"=FALSE, "Boolean 60"=FALSE, "Boolean 61"=FALSE, "Boolean 62"=FALSE, "Boolean 63"=FALSE, "Boolean 64"=FALSE, "Boolean 65"=FALSE, "Boolean 66"=FALSE, "Boolean 67"=FALSE, "Boolean 68"=FALSE, "Boolean 69"=FALSE, "Boolean 70"=FALSE, "Boolean 71"=FALSE, "Boolean 72"=FALSE, "Boolean 73"=FALSE, "Boolean 74"=FALSE, "Boolean 75"=FALSE, "Boolean 76"=FALSE, "Boolean 77"=FALSE, "Boolean 78"=FALSE, "Boolean 79"=FALSE, "Boolean 80"=FALSE, "Boolean 81"=FALSE, "Boolean 82"=FALSE, "Boolean 83"=FALSE, "Boolean 84"=FALSE, "Boolean 85"=FALSE, "Boolean 86"=FALSE, "Boolean 87"=FALSE, "Boolean 88"=FALSE, "Boolean 89"=FALSE, "Boolean 90"=FALSE, "Boolean 91"=FALSE, "Boolean 92"=FALSE, "Boolean 93"=FALSE, "Boolean 94"=FALSE, "Boolean 95"=FALSE, "Boolean 96"=FALSE, "Boolean 97"=FALSE, "Boolean 98"=FALSE, "Boolean 99"=FALSE, "Boolean 100"=FALSE}], "PresetClust.Clear"=FALSE ("AdjClust.ClearTable"), "Sel"=w2395) -> (w2386:T9)
            n2205 = call "FeedbackDecode_UpdatePresetsTable.vi"("StimClustIn"=w2386) -> ("StimClustOut"=w2385:T9)  [unwired: 2 in]
            n2206 = local read "LoopCnt"() -> (w2407:u64)
            n2207 = call "FeedbackDecode_UpdateParamsTable.vi"("StimClustIn"=w2385) -> ("StimClustOut"=w2397:T9)  [unwired: 2 in]
            n2208 = call "FeedbackDecode_Params2UEA.vi"("StimClustIn"=w2397) -> ("StimClustOut"=w2398:T9)  [unwired: 2 in]
            n2209 = Format Into String(w2407) -> (resulting string=w2399:string)  [unwired: 3 in, 1 out]
            n2210 = local read "NIPTime"() -> (w2403:dbl)
            n2211 = call "FeedbackDecode_BuildStimCmd.vi"("EncodeClustIn"=w2398) -> ("EncodeClustOut"=w2413:T9, "StimCmd"=w2387:string)  [unwired: 1 in]
            n2212 = local read "EventParamsFID"() -> (w2411:refnum<file>)
            n2213 = Concatenate Strings("ClearPresets:SS.EventID=" ("string"), w2399) -> (w2406:string)
            n2214 = call-poly "FeedbackDecode_VariablesToString.vi"("Format"="%0.0f", "ValueIn"=w2403, "FieldName"="NIPTime" ("Key Word")) -> ("StringOut"=w2400:string)  [unwired: 4 in]
            n2215 = local read "DecodeClust"() -> (w2412:T5)
            n2216 = Concatenate Strings(w2406, ";", w2387, w2400) -> (w2405:string)
            n2217 = call "FeedbackDecode_WriteTextEOL.vi"("text"=w2405, "refnum in"=w2411) -> ()  [unwired: 8 in, 2 out]
            n2218 = Bundle By Name(cluster=w2412, "EventStr"=w2405) -> (w2404:T5)
            n2219 = local write "StimCmd"(w2387) -> ()
            n2220 = local write "EncodeClust"(w2413) -> ()
            n2221 = call "FeedbackDecode_MLComCtrl.vi"("DecodeClustIn"=w2404, "Mode"=T19."SendEvent") -> ()  [unwired: 6 in, 4 out]
          }
          event Value Change {
            n2222 = event-data() -> ()  [unwired: 1 in, 6 out]
            n2223 = local read "EncodeClust"() -> (w2423:T9)
            n2224 = Bundle By Name(cluster=w2423, "Stim"=FALSE) -> (w2421:T9)
            n2225 = call "FeedbackDecode_BuildStimCmd.vi"("EncodeClustIn"=w2421) -> ("EncodeClustOut"=w2433:T9, "StimCmd"=w2415:string)  [unwired: 1 in]
            n2226 = local read "LoopCnt"() -> (w2427:u64)
            n2227 = local read "NIPTime"() -> (w2420:dbl)
            n2228 = local write "EncodeClust"(w2433) -> ()
            n2229 = local write "StimCmd"(w2415) -> ()
            n2230 = Format Into String(w2427) -> (resulting string=w2416:string)  [unwired: 3 in, 1 out]
            n2231 = call-poly "FeedbackDecode_VariablesToString.vi"("Format"="%0.0f", "ValueIn"=w2420, "FieldName"="NIPTime" ("Key Word")) -> ("StringOut"=w2417:string)  [unwired: 4 in]
            n2232 = local read "EventParamsFID"() -> (w2431:refnum<file>)
            n2233 = Concatenate Strings("ChangeStimMode:SS.EventID=" ("string"), w2416) -> (w2426:string)
            n2234 = local read "DecodeClust"() -> (w2432:T5)
            n2235 = Concatenate Strings(w2426, ";", w2415, w2417) -> (w2425:string)
            n2236 = call "FeedbackDecode_WriteTextEOL.vi"("text"=w2425, "refnum in"=w2431) -> ()  [unwired: 8 in, 2 out]
            n2237 = Bundle By Name(cluster=w2432, "EventStr"=w2425) -> (w2424:T5)
            n2238 = call "FeedbackDecode_MLComCtrl.vi"("DecodeClustIn"=w2424, "Mode"=T19."SendEvent") -> ()  [unwired: 6 in, 4 out]
          }
          event Value Change {
            n2239 = event-data() -> ("NewVal"=w2435:bool)  [unwired: 1 in, 5 out]
            n2240 = case shown="True" w2435 {
              frame False {
                n2241 = local write "PulseStim"(FALSE ("PulseStim")) -> ()
                n2242 = local write "BaseCnt3"(-inf) -> ()
                n2243 = local read "EncodeClust"() -> (w2454:T9)
                n2244 = local read "LoopCnt"() -> (w2448:u64)
                n2245 = call "FeedbackDecode_BuildStimCmd.vi"("EncodeClustIn"=w2454) -> ("EncodeClustOut"=w2453:T9, "StimCmd"=w2437:string)  [unwired: 1 in]
                n2246 = local read "NIPTime"() -> (w2444:dbl)
                n2247 = Format Into String(w2448) -> (resulting string=w2440:string)  [unwired: 3 in, 1 out]
                n2248 = local write "EncodeClust"(w2453) -> ()
                n2249 = local read "EventParamsFID"() -> (w2451:refnum<file>)
                n2250 = Concatenate Strings("ManualStim:SS.EventID=" ("string"), w2440, ";" ("string")) -> (w2447:string)
                n2251 = call-poly "FeedbackDecode_VariablesToString.vi"("Format"="%0.0f", "ValueIn"=w2444, "FieldName"="NIPTime" ("Key Word")) -> ("StringOut"=w2441:string)  [unwired: 4 in]
                n2252 = local write "StimCmd"(w2437) -> ()
                n2253 = Concatenate Strings(w2447, "SS.PulseStim=0;" ("string"), w2437, w2441) -> (w2446:string)
                n2254 = local read "DecodeClust"() -> (w2452:T5)
                n2255 = call "FeedbackDecode_WriteTextEOL.vi"("text"=w2446, "refnum in"=w2451) -> ()  [unwired: 8 in, 2 out]
                n2256 = Bundle By Name(cluster=w2452, "EventStr"=w2446) -> (w2445:T5)
                n2257 = call "FeedbackDecode_MLComCtrl.vi"("DecodeClustIn"=w2445, "Mode"=T19."SendEvent") -> ()  [unwired: 6 in, 4 out]
              }
              frame True {
                n2258 = local read "EncodeClust"() -> (w2460:T9)
                n2259 = local write "PulseStim"(FALSE ("PulseStim")) -> ()
                n2260 = Unbundle By Name(w2460) -> ("Train Period"=w2461:dbl)
                n2261 = local read "EncodeClust"() -> (w2479:T9)
                n2262 = local read "LoopCnt"() -> (w2458:u64)
                n2263 = expression code="x*100"(w2461) -> (w2459:dbl)
                n2264 = local read "LoopCnt"() -> (w2473:u64)
                n2265 = Add(x=w2458, y=w2459) -> (x+y=w2457:dbl)
                n2266 = call "FeedbackDecode_BuildStimCmd.vi"("EncodeClustIn"=w2479) -> ("EncodeClustOut"=w2478:T9, "StimCmd"=w2462:string)  [unwired: 1 in]
                n2267 = local write "BaseCnt3"(w2457) -> ()
                n2268 = local read "NIPTime"() -> (w2469:dbl)
                n2269 = Format Into String(w2473) -> (resulting string=w2465:string)  [unwired: 3 in, 1 out]
                n2270 = local write "EncodeClust"(w2478) -> ()
                n2271 = Concatenate Strings("ManualStim:SS.EventID=" ("string"), w2465, ";" ("string")) -> (w2472:string)
                n2272 = call-poly "FeedbackDecode_VariablesToString.vi"("Format"="%0.0f", "ValueIn"=w2469, "FieldName"="NIPTime" ("Key Word")) -> ("StringOut"=w2466:string)  [unwired: 4 in]
                n2273 = local read "EventParamsFID"() -> (w2476:refnum<file>)
                n2274 = local write "StimCmd"(w2462) -> ()
                n2275 = Concatenate Strings(w2472, "SS.PulseStim=1;" ("string"), w2462, w2466) -> (w2471:string)
                n2276 = local read "DecodeClust"() -> (w2477:T5)
                n2277 = call "FeedbackDecode_WriteTextEOL.vi"("text"=w2471, "refnum in"=w2476) -> ()  [unwired: 8 in, 2 out]
                n2278 = Bundle By Name(cluster=w2477, "EventStr"=w2471) -> (w2470:T5)
                n2279 = call "FeedbackDecode_MLComCtrl.vi"("DecodeClustIn"=w2470, "Mode"=T19."SendEvent") -> ()  [unwired: 6 in, 4 out]
              }
            }
          }
          event Value Change {
            n2280 = event-data() -> ()  [unwired: 1 in, 6 out]
            n2281 = local read "EncodeClust"() -> (w2497:T9)
            n2282 = call "FeedbackDecode_BuildStimCmd.vi"("EncodeClustIn"=w2497) -> ("EncodeClustOut"=w2496:T9, "StimCmd"=w2481:string)  [unwired: 1 in]
            n2283 = local read "LoopCnt"() -> (w2491:u64)
            n2284 = local write "EncodeClust"(w2496) -> ()
            n2285 = local read "NIPTime"() -> (w2487:dbl)
            n2286 = Format Into String(w2491) -> (resulting string=w2482:string)  [unwired: 3 in, 1 out]
            n2287 = call-poly "FeedbackDecode_VariablesToString.vi"("Format"="%0.0f", "ValueIn"=w2487, "FieldName"="NIPTime" ("Key Word")) -> ("StringOut"=w2484:string)  [unwired: 4 in]
            n2288 = local read "EventParamsFID"() -> (w2494:refnum<file>)
            n2289 = Concatenate Strings("ChangeStimStep:SS.EventID=" ("string"), w2482) -> (w2490:string)
            n2290 = local write "StimCmd"(w2481) -> ()
            n2291 = local read "DecodeClust"() -> (w2495:T5)
            n2292 = Concatenate Strings(w2490, ";", w2481, w2484) -> (w2489:string)
            n2293 = call "FeedbackDecode_WriteTextEOL.vi"("text"=w2489, "refnum in"=w2494) -> ()  [unwired: 8 in, 2 out]
            n2294 = Bundle By Name(cluster=w2495, "EventStr"=w2489) -> (w2488:T5)
            n2295 = call "FeedbackDecode_MLComCtrl.vi"("DecodeClustIn"=w2488, "Mode"=T19."SendEvent") -> ()  [unwired: 6 in, 4 out]
          }
          event Value Change {
            n2296 = event-data() -> ()  [unwired: 1 in, 6 out]
            n2297 = local read "EncodeClust"() -> (w2515:T9)
            n2298 = call "FeedbackDecode_BuildStimCmd.vi"("EncodeClustIn"=w2515) -> ("EncodeClustOut"=w2514:T9, "StimCmd"=w2499:string)  [unwired: 1 in]
            n2299 = local read "LoopCnt"() -> (w2509:u64)
            n2300 = local write "EncodeClust"(w2514) -> ()
            n2301 = local read "NIPTime"() -> (w2505:dbl)
            n2302 = Format Into String(w2509) -> (resulting string=w2500:string)  [unwired: 3 in, 1 out]
            n2303 = call-poly "FeedbackDecode_VariablesToString.vi"("Format"="%0.0f", "ValueIn"=w2505, "FieldName"="NIPTime" ("Key Word")) -> ("StringOut"=w2502:string)  [unwired: 4 in]
            n2304 = local read "EventParamsFID"() -> (w2512:refnum<file>)
            n2305 = Concatenate Strings("ChangeJitter:SS.EventID=" ("string"), w2500) -> (w2508:string)
            n2306 = local write "StimCmd"(w2499) -> ()
            n2307 = Concatenate Strings(w2508, ";", w2499, w2502) -> (w2507:string)
            n2308 = local read "DecodeClust"() -> (w2513:T5)
            n2309 = call "FeedbackDecode_WriteTextEOL.vi"("text"=w2507, "refnum in"=w2512) -> ()  [unwired: 8 in, 2 out]
            n2310 = Bundle By Name(cluster=w2513, "EventStr"=w2507) -> (w2506:T5)
            n2311 = call "FeedbackDecode_MLComCtrl.vi"("DecodeClustIn"=w2506, "Mode"=T19."SendEvent") -> ()  [unwired: 6 in, 4 out]
          }
          event Value Change {
            n2312 = event-data() -> ()  [unwired: 1 in, 6 out]
            n2313 = local read "EncodeClust"() -> (w2533:T9)
            n2314 = call "FeedbackDecode_BuildStimCmd.vi"("EncodeClustIn"=w2533) -> ("EncodeClustOut"=w2532:T9, "StimCmd"=w2517:string)  [unwired: 1 in]
            n2315 = local read "LoopCnt"() -> (w2527:u64)
            n2316 = local write "EncodeClust"(w2532) -> ()
            n2317 = local read "NIPTime"() -> (w2523:dbl)
            n2318 = Format Into String(w2527) -> (resulting string=w2518:string)  [unwired: 3 in, 1 out]
            n2319 = call-poly "FeedbackDecode_VariablesToString.vi"("Format"="%0.0f", "ValueIn"=w2523, "FieldName"="NIPTime" ("Key Word")) -> ("StringOut"=w2520:string)  [unwired: 4 in]
            n2320 = Concatenate Strings("ChangeBFreq:SS.EventID=" ("string"), w2518) -> (w2526:string)
            n2321 = local read "EventParamsFID"() -> (w2530:refnum<file>)
            n2322 = local write "StimCmd"(w2517) -> ()
            n2323 = Concatenate Strings(w2526, ";", w2517, w2520) -> (w2525:string)
            n2324 = local read "DecodeClust"() -> (w2531:T5)
            n2325 = call "FeedbackDecode_WriteTextEOL.vi"("text"=w2525, "refnum in"=w2530) -> ()  [unwired: 8 in, 2 out]
            n2326 = Bundle By Name(cluster=w2531, "EventStr"=w2525) -> (w2524:T5)
            n2327 = call "FeedbackDecode_MLComCtrl.vi"("DecodeClustIn"=w2524, "Mode"=T19."SendEvent") -> ()  [unwired: 6 in, 4 out]
          }
          event Value Change {
            n2328 = event-data() -> ()  [unwired: 1 in, 6 out]
            n2329 = local read "EncodeClust"() -> (w2551:T9)
            n2330 = call "FeedbackDecode_BuildStimCmd.vi"("EncodeClustIn"=w2551) -> ("EncodeClustOut"=w2550:T9, "StimCmd"=w2535:string)  [unwired: 1 in]
            n2331 = local read "LoopCnt"() -> (w2545:u64)
            n2332 = local write "EncodeClust"(w2550) -> ()
            n2333 = local read "NIPTime"() -> (w2541:dbl)
            n2334 = Format Into String(w2545) -> (resulting string=w2536:string)  [unwired: 3 in, 1 out]
            n2335 = call-poly "FeedbackDecode_VariablesToString.vi"("Format"="%0.0f", "ValueIn"=w2541, "FieldName"="NIPTime" ("Key Word")) -> ("StringOut"=w2538:string)  [unwired: 4 in]
            n2336 = local read "EventParamsFID"() -> (w2548:refnum<file>)
            n2337 = Concatenate Strings("ChangeBAmp:SS.EventID=" ("string"), w2536) -> (w2544:string)
            n2338 = local write "StimCmd"(w2535) -> ()
            n2339 = local read "DecodeClust"() -> (w2549:T5)
            n2340 = Concatenate Strings(w2544, ";", w2535, w2538) -> (w2543:string)
            n2341 = call "FeedbackDecode_WriteTextEOL.vi"("text"=w2543, "refnum in"=w2548) -> ()  [unwired: 8 in, 2 out]
            n2342 = Bundle By Name(cluster=w2549, "EventStr"=w2543) -> (w2542:T5)
            n2343 = call "FeedbackDecode_MLComCtrl.vi"("DecodeClustIn"=w2542, "Mode"=T19."SendEvent") -> ()  [unwired: 6 in, 4 out]
          }
          event "TASKA Shared Control": Value Change {
            n2344 = event-data() -> ("NewVal"=w2555:bool)  [unwired: 1 in, 5 out]
            n2345 = case shown="True" w2555 {
              tunnel: [0.0 1.0] -> w2554
              frame False {
              }
              frame True {
              }
            }
            n2346 = local read "LoopCnt"() -> (w2564:u64)
            n2347 = call-poly "FeedbackDecode_VariablesToString.vi"("Format"="%d", "ValueIn"=w2554, "FieldName"="TASKASensors.SharedControl.Ready") -> ("StringOut"=w2571:string)  [unwired: 4 in]
            n2348 = local read "NIPTime"() -> (w2560:dbl)
            n2349 = Format Into String(w2564) -> (resulting string=w2556:string)  [unwired: 3 in, 1 out]
            n2350 = local read "EventParamsFID"() -> (w2568:refnum<file>)
            n2351 = local read "DecodeClust"() -> (w2569:T5)
            n2352 = Concatenate Strings("SharedControl:SS.EventID=" ("string"), w2556) -> (w2563:string)
            n2353 = call-poly "FeedbackDecode_VariablesToString.vi"("Format"="%0.0f", "ValueIn"=w2560, "FieldName"="NIPTime" ("Key Word")) -> ("StringOut"=w2557:string)  [unwired: 4 in]
            n2354 = Concatenate Strings(w2563, ";", w2571, w2557) -> (w2562:string)
            n2355 = call "FeedbackDecode_WriteTextEOL.vi"("text"=w2562, "refnum in"=w2568) -> ()  [unwired: 8 in, 2 out]
            n2356 = Bundle By Name(cluster=w2569, "EventStr"=w2562) -> (w2561:T5)
            n2357 = call "FeedbackDecode_MLComCtrl.vi"("DecodeClustIn"=w2561, "Mode"=T19."SendEvent") -> ()  [unwired: 6 in, 4 out]
          }
          event "TASKA Timer": Value Change {
            n2358 = event-data() -> ("NewVal"=w2575:bool)  [unwired: 1 in, 5 out]
            n2359 = case shown="True" w2575 {
              frame True {
                n2360 = local read "LoopCnt"() -> (w2580:u64)
                n2361 = local read "NIPTime"() -> (w2583:dbl)
                n2362 = Format Into String(w2580) -> (resulting string=w2587:string)  [unwired: 3 in, 1 out]
                n2363 = local read "EventParamsFID"() -> (w2577:refnum<file>)
                n2364 = Concatenate Strings("SharedControlStartTime:SS.EventID=" ("string"), w2587) -> (w2581:string)
                n2365 = call-poly "FeedbackDecode_VariablesToString.vi"("Format"="%0.0f", "ValueIn"=w2583, "FieldName"="NIPTime" ("Key Word")) -> ("StringOut"=w2586:string)  [unwired: 4 in]
                n2366 = Concatenate Strings(w2581, ";", w2586) -> (w2582:string)
                n2367 = call "FeedbackDecode_WriteTextEOL.vi"("text"=w2582, "refnum in"=w2577) -> ()  [unwired: 8 in, 2 out]
